vi "Split 16xI16 to 1xI16.vi"(0 "data in":i16[](array[numeric])=[0, 0, 0, 0, 0, 0, 0, 0, 0, 0, 0, 0, 0, 0, 0, 0], 2 "reset":bool, 5 "input valid":bool, 12 "ready for output (T)":bool=TRUE) -> (4 "data out":i16, 6 "output valid":bool, 14 "ready for input":bool)   [LabVIEW 2018, in "Streaming FPGA.lvlib"]
doc: "Splits an array of 16 I16 elements to I16 elements. One data input generates 16 data outputs."
uses:
  Streaming FPGA.lvlib
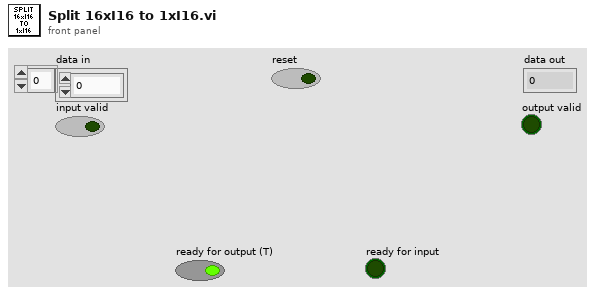
[diagram p1: front panel]
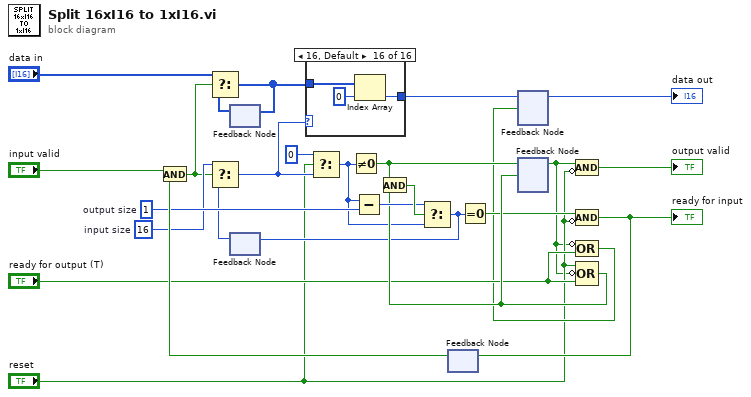
[diagram p0: block diagram]
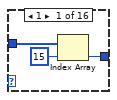
[diagram p2: hidden frame]
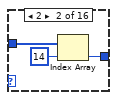
[diagram p3: hidden frame]
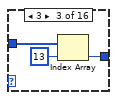
[diagram p4: hidden frame]
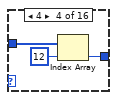
[diagram p5: hidden frame]
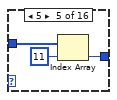
[diagram p6: hidden frame]
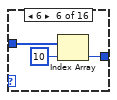
[diagram p7: hidden frame]
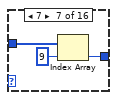
[diagram p8: hidden frame]
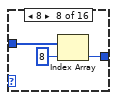
[diagram p9: hidden frame]
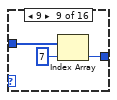
[diagram p10: hidden frame]
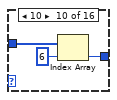
[diagram p11: hidden frame]
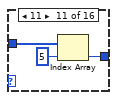
[diagram p12: hidden frame]
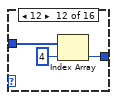
[diagram p13: hidden frame]
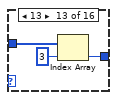
[diagram p14: hidden frame]
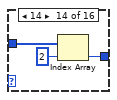
[diagram p15: hidden frame]
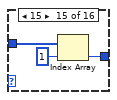
[diagram p16: hidden frame]
diagram:
  w22 = u16 1  # output size
  w10 = u16 16  # input size
  n1 = feedback #1() -> (w13:i16[])  [unwired: 1 in]
  n2 = feedback #2() -> (w20:u16)  [unwired: 1 in]
  n3 = feedback #3() -> (w26:bool)  [unwired: 1 in]
  n4 = And(x="input valid", y=w26) -> (x .and. y?=w8:bool)
  n5 = Select(t="data in", s=w8, f=w13) -> (s? t:f=w12:i16[])
  n6 = Select(t=w10, s=w8, f=w20) -> (s? t:f=w16:u16)
  n7 = feedback-in #1(w12) -> ()
  n8 = case shown="16, Default" w16 {
    tunnel: w12 -> [w29 w32 w35 w38 w41 w44 w47 w50 w53 w56 w59 w62 w65 w68 w71 w74]
    tunnel: [w27 w30 w33 w36 w39 w42 w45 w48 w51 w54 w57 w60 w63 w66 w69 w72] -> w25
    frame 1 {
      n9 = Index Array(array=w29, index=15) -> (element=w27:i16)
    }
    frame 2 {
      n10 = Index Array(array=w32, index=14) -> (element=w30:i16)
    }
    frame 3 {
      n11 = Index Array(array=w35, index=13) -> (element=w33:i16)
    }
    frame 4 {
      n12 = Index Array(array=w38, index=12) -> (element=w36:i16)
    }
    frame 5 {
      n13 = Index Array(array=w41, index=11) -> (element=w39:i16)
    }
    frame 6 {
      n14 = Index Array(array=w44, index=10) -> (element=w42:i16)
    }
    frame 7 {
      n15 = Index Array(array=w47, index=9) -> (element=w45:i16)
    }
    frame 8 {
      n16 = Index Array(array=w50, index=8) -> (element=w48:i16)
    }
    frame 9 {
      n17 = Index Array(array=w53, index=7) -> (element=w51:i16)
    }
    frame 10 {
      n18 = Index Array(array=w56, index=6) -> (element=w54:i16)
    }
    frame 11 {
      n19 = Index Array(array=w59, index=5) -> (element=w57:i16)
    }
    frame 12 {
      n20 = Index Array(array=w62, index=4) -> (element=w60:i16)
    }
    frame 13 {
      n21 = Index Array(array=w65, index=3) -> (element=w63:i16)
    }
    frame 14 {
      n22 = Index Array(array=w68, index=2) -> (element=w66:i16)
    }
    frame 15 {
      n23 = Index Array(array=w71, index=1) -> (element=w69:i16)
    }
    frame 16, Default {
      n24 = Index Array(array=w74, index=0) -> (element=w72:i16)
    }
  }
  n25 = Select(t=u16 0, s="reset", f=w16) -> (s? t:f=w14:u16)
  n26 = Not Equal To 0?(x=w14) -> (x != 0?=w24:bool)
  n27 = Subtract(x=w14, y=w22) -> (x-y=w21:u16)
  n28 = feedback #4() -> (→"data out":i16)  [unwired: 1 in]
  n29 = feedback #5() -> (w1:bool)  [unwired: 1 in]
  n30 = Compound Arithmetic op=AND(w1, invert "reset") -> (→"output valid":bool)
  n31 = Compound Arithmetic op=OR(invert w1, "ready for output (T)") -> (w3:bool)
  n32 = feedback-in #4(w25, w3) -> ()
  n33 = Compound Arithmetic op=OR("reset", invert w1, "ready for output (T)") -> (w19:bool)
  n34 = And(x=w24, y=w19) -> (x .and. y?=w23:bool)
  n35 = Select(t=w21, s=w23, f=w14) -> (s? t:f=w18:u16)
  n36 = feedback-in #2(w18) -> ()
  n37 = Equal To 0?(x=w18) -> (x = 0?=w17:bool)
  n38 = feedback-in #5(w24, w19) -> ()
  n39 = Compound Arithmetic op=AND(w17, invert "reset") -> (w6:bool)
  "ready for input" <- w6
  n40 = feedback-in #3(w6) -> ()
